vi "IFwHostTest.vi"() -> ()   [LabVIEW 2017]
uses:
  <vilib>/rvi/interface/nirviOpenFPGA/nirviOpenFPGA.xnode
  <instrlib>/_niInstr/Instruction Framework/v1/Host/Instruction Target/niInstr Instruction Target v1 Host.lvclass
  <instrlib>/_niInstr/FIFO Register Bus/v1/Host/niInstr FIFO Register Bus v1 Host.lvclass
  <instrlib>/_niInstr/Instruction Framework/v1/Host/Subsystem Map/niInstr Subsystem Map v1 Host.lvclass
  <instrlib>/_niInstr/Instruction Framework/v1/Host/Subsystem Map/Private/Lookup Single Context.vi
  <vilib>/rvi/interface/nirviCloseFPGA/nirviCloseFPGA.xnode
  <vilib>/FPGAPlugInAG/Dynamic/niLvFpga_Close_Dynamic.vi
  <vilib>/rvi/interface/nirviReadWriteControl/nirviReadWriteControl.xnode
  NiFpgaLv.dll
  <vilib>/Utility/error.llb/Error Cluster From Error Code.vi
  <vilib>/rvi/interface/Simulation/niFpgaSimulationCallBeginRW.vi
  <vilib>/rvi/errors/niLvFpgaAdjustHostInterfaceError.vi
  FPGA/IFwTest.vi
  C:/Program Files (x86)/National Instruments/LabVIEW 2017/instr.lib/_niInstr/Instruction Framework/v1/Host/Instruction Target/niInstr Instruction Target v1 Host.lvclass
panel:
  out "perturbAmp":sgl
  out "manualInput":sgl
  out "rampRate":sgl
  out "numOfInterleaves":u8
  in  "address":u64
  in  "data":u64 format="%.0x"
  out "SGL 2":sgl
  in  "set":bool
  in  "stop":bool
  in  "SGL":sgl format="%#_13g"
  out "U32":u32 format="%.0x"
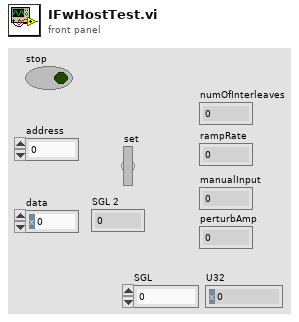
[diagram p1: front panel]
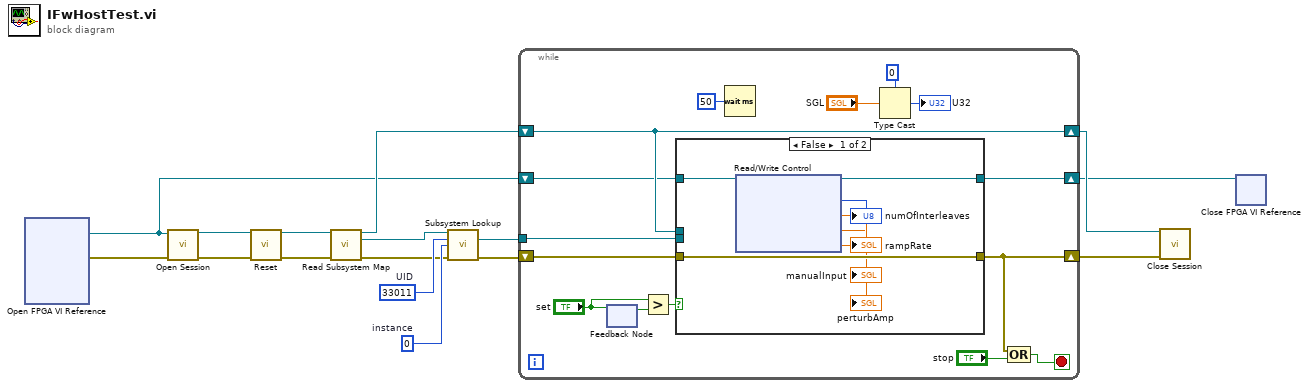
[diagram p0: block diagram]
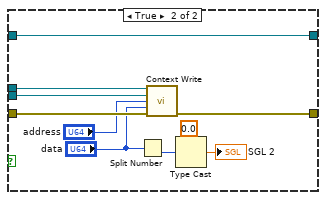
[diagram p2: hidden frame]
diagram:
  w13 = u8 0  # instance
  w14 = u16 33011  # UID
  n1 = xnode "Open FPGA VI Reference"() -> ("FPGA VI Reference Out"=w2:refnum<k20>, "error out"=w3:errorcluster)  [unwired: 2 in]
  n2 = call <instrlib>:"Open Session.vi"("fpga ref"=w2, "error in"=w3) -> ("session out"=w9:refnum<class "niInstr FIFO Register Bus v1 Host.lvclass">, "error out"=w10:errorcluster)  [unwired: 12 in]
  n3 = call-dynamic "Reset.vi"("session in"=w9, "error in"=w10) -> ("session out"=w7:refnum<class "niInstr FIFO Register Bus v1 Host.lvclass">, "error out"=w8:errorcluster)  [unwired: 12 in]
  n4 = call <instrlib>:"Read Subsystem Map.vi"("instruction target in"=w7, "error in"=w8) -> ("instruction target out"=w6:refnum<class "niInstr FIFO Register Bus v1 Host.lvclass">, "subsystem map"=w5:refnum<class "niInstr Subsystem Map v1 Host.lvclass">, "error out"=w4:errorcluster)  [unwired: 11 in]
  n5 = call-poly <instrlib>:"Subsystem Lookup.vi"("subsystem map in"=w5, "UID"=w14, "instance"=w13, "error in"=w4) -> ("context"=w12:refnum<class "niInstr Instruction Framework Context v1 Host.lvclass">, "error out"=w11:errorcluster)  [unwired: 8 in, 2 out]
  n6 = while {
    shift-right: [w31] -> w16
    shift-left: w6 -> [w31]
    tunnel: w12 -> [w29]
    shift-right: [w22] -> w15
    shift-left: w11 -> [w30]
    shift-right: [w20] -> w1
    shift-left: w2 -> [w24]
    stop <- w21 stop-if-true
    n7 = feedback-in #1("set") -> ()
    n8 = feedback #1() -> (w28:bool)  [unwired: 1 in]
    n9 = Greater?(x="set", y=w28) -> (0:w26:bool)
    n10 = case shown="False" w26 {
      tunnel: w31 -> [_ w48]
      tunnel: w30 -> [w37 w47]
      tunnel: w29 -> [_ w46]
      tunnel: [w37 w45] -> w22
      tunnel: w24 -> [w38 w43]
      tunnel: [w36 w43] -> w20
      frame False {
        n11 = xnode "Read/Write Control"("FPGA VI Reference In"=w38) -> ("FPGA VI Reference Out"=w36:refnum<k20>, "numOfInterleaves"=→"numOfInterleaves":u8, "rampRate"=→"rampRate":sgl, "manualInput"=→"manualInput":sgl, "perturbAmp"=→"perturbAmp":sgl)  [unwired: 1 in, 1 out]
      }
      frame True {
        n12 = Split Number(x="data") -> (lo(x)=w41:u32)  [unwired: 1 out]
        n13 = call <instrlib>:"Context Write.vi"("instruction target in"=w48, "context in"=w46, "address"="address", "data"="data", "error in"=w47) -> ("error out"=w45:errorcluster)  [unwired: 8 in, 2 out]
        n14 = Type Cast(type=sgl 0.0, x=w41) -> (*(type *) &x=→"SGL 2":sgl)
      }
    }
    n15 = Wait (ms)(milliseconds to wait=u32 50) -> ()  [unwired: 1 out]
    n16 = Type Cast(type=u32 0, x="SGL") -> (*(type *) &x=→"U32":u32)
    n17 = Compound Arithmetic op=OR(w22, "stop") -> (w21:bool)
  }
  n18 = call-dynamic "Close Session.vi"("session in"=w16, "error in"=w15) -> ()  [unwired: 13 in, 1 out]
  n19 = xnode "Close FPGA VI Reference"("FPGA VI Reference In"=w1) -> ()  [unwired: 1 in, 1 out]
